vi "dt with overflow.vi"(10 "t0":u32, 11 "t1":u32) -> (3 "t1-t0":u32)   [LabVIEW 2012]
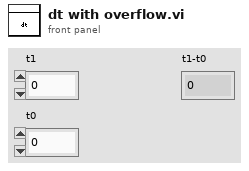
[diagram p1: front panel]
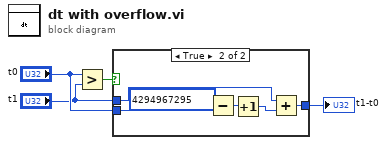
[diagram p0: block diagram]
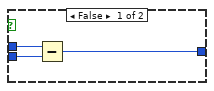
[diagram p2: hidden frame]
diagram:
  n1 = Greater?(x="t0", y="t1") -> (0:w1:bool)
  n2 = case shown="True" w1 {
    tunnel: "t1" -> [w7 w9]
    tunnel: "t0" -> [w6 w10]
    tunnel: [w5 w8] -> w2
    frame False {
      n3 = Subtract(x=w7, y=w6) -> (x-y=w5:u32)
    }
    frame True {
      n4 = Subtract(x=u32 4294967295, y=w10) -> (x-y=w12:u32)
      n5 = Increment(x=w12) -> (x+1=w11:u32)
      n6 = Add(x=w9, y=w11) -> (x+y=w8:u32)
    }
  }
  "t1-t0" <- w2
